vi "Theme Info Entry Enum To String.vi"(11 "Theme Info Entry":T1) -> (3 "Root Theme Entry String":string)   [LabVIEW 2021, in "Appearance Actor.lvlib" / "Generic Theme.lvclass"]
doc: "Converts <B>Theme Info Entry</B> enum into String."
uses:
  Generic Theme.lvclass
  Typedefs/Theme Info Entry--enum.ctl
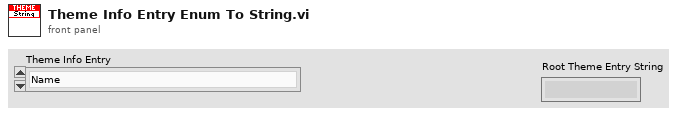
[diagram p1: front panel]
types:
  T1 = typedef "Appearance Actor.lvlib/Generic Theme.lvclass/Theme Info Entry--enum.ctl" = enum16{"Name", "Type", "Version"}
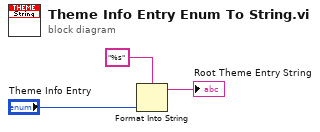
[diagram p0: block diagram]
diagram:
  n1 = Format Into String(format string="%s", "Theme Info Entry") -> (resulting string=→"Root Theme Entry String":string)  [unwired: 2 in, 1 out]
